vi "Add Response to BST.vi"(6 "JSON Value in":variant, 7 "error":bool, 8 "error in (no error)":errorcluster, 9 "id value":string, 10 "jsonrpc":string="2.0", 11 "Server in":refnum<class "JSONRPC Server.lvclass">) -> (0 "error out":errorcluster, 1 "response string":string, 2 "replaced":bool, 3 "Server out":refnum<class "JSONRPC Server.lvclass">)   [LabVIEW 2020, in "JSON-RPC Lib.lvlib" / "JSONRPC Server.lvclass"]
uses:
  JSONRPC Server.lvclass
  Get Response Tree.vi
  Response/Response.lvclass
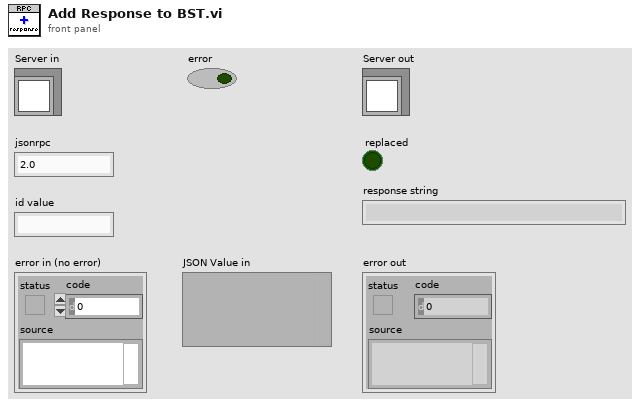
[diagram p1: front panel]
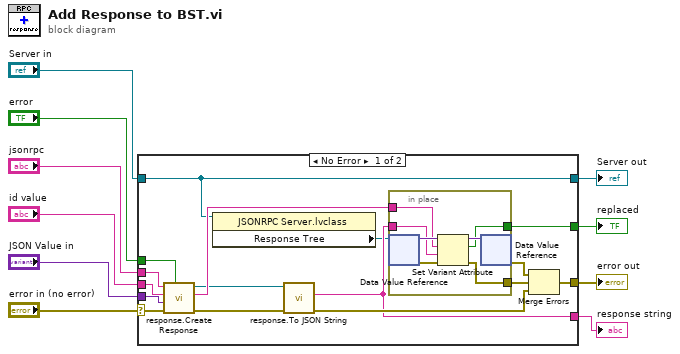
[diagram p0: block diagram]
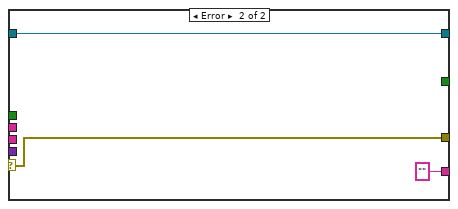
[diagram p2: hidden frame]
diagram:
  n1 = case shown="No Error" "error in (no error)" {
    selector: "error in (no error)" -> [w26 w36]
    tunnel: [w21 w36] -> w9
    tunnel: [w12 w35] -> w7
    tunnel: "Server in" -> [w12 w35]
    tunnel: "JSON Value in" -> [w19 _]
    tunnel: "error" -> [w20 _]
    tunnel: [w24 _] -> w4
    tunnel: "jsonrpc" -> [w18 _]
    tunnel: "id value" -> [w17 _]
    tunnel: [w13 "" ("JSON String")] -> w1
    frame No Error {
      n2 = call "response.Create Response.vi"("error"=w20, "error in (no error)"=w26, "JSON Value in"=w19, "id value"=w17, "jsonrpc"=w18) -> ("error out"=w15:errorcluster, "id String"=w25:string, "Response out"=w16:refnum<class "Response.lvclass">)  [unwired: 4 in]
      n3 = property class="JSONRPC Server.lvclass"(reference=w12) -> ("Response Tree"=w11:refnum<data-value>)  [unwired: 1 in, 2 out]
      n4 = call "response.To JSON String.vi"("error in (no error)"=w15, "Response in"=w16) -> ("error out"=w14:errorcluster, "JSON String"=w13:string)  [unwired: 7 in, 1 out]
      n5 = in-place {
        in-place-border: w25 -> [w31]
        in-place-border: w13 -> [w30]
        in-place-border: [w29] -> w24
        in-place-border: [w27] -> w22
        n6 = in-place-dvr #1(w11) -> (w33:variant, w28:errorcluster)
        n7 = Set Variant Attribute(Variant=w33, name=w31, value=w30, error in=w28) -> (Variant out=w32:variant, replaced=w29:bool, error out=w27:errorcluster)
        n8 = in-place-dvr #1(w32) -> (w23:errorcluster)  [unwired: 1 out]
      }
      n9 = Merge Errors(w23, w22, w14) -> (w21:errorcluster)
    }
    frame Error {
    }
  }
  "error out" <- w9
  "Server out" <- w7
  "replaced" <- w4
  "response string" <- w1
